vi "LCP_Scale.vi"() -> ()   [LabVIEW 2019]
uses:
  <vilib>/Instr/_visa.llb/VISA Configure Serial Port (Instr).vi
  <vilib>/Utility/file.llb/Write Delimited Spreadsheet (DBL).vi
panel:
  in  "Boolean":bool
  in  ".CSV filename":path
  in  "Weight Name":string
  out "Weight":string
  in  "stop":bool
  in  "Weights Number":i32
  in  "Ring":u8(ring) items=["Send data", "Activate calibration function", "Activate counting function", "Weighing unit selection", "Taring"]
  in  "VISA resource port":refnum<visa-resource-name>
  # ".CSV FILE NAME"
  # "VISA PORT"
  # "INSTRUCTION"
  # "REFERENCE WEIGHTS NUMBER"
  # "REFERENCE WEIGHT NAME"
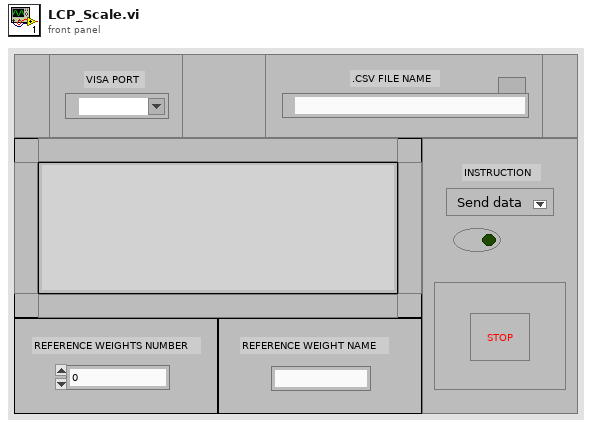
[diagram p1: front panel]
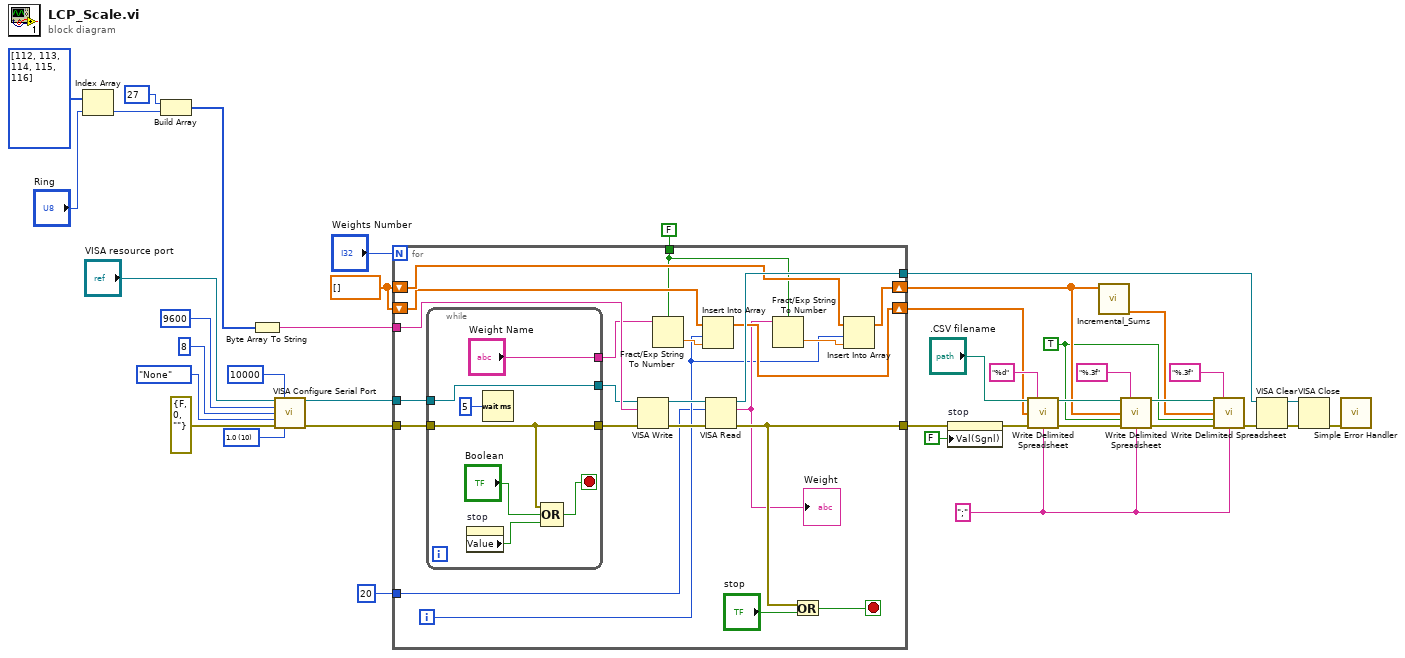
[diagram p0: block diagram]
diagram:
  w11 = TRUE ("append to file? (new file:F)")
  w8 = ";" ("delimiter (\\t)")
  w20 = dbl[] []
  w34 = u16 10 items=["1.0"=10, "1.5"=15, "2.0"=20] ("stop bits (10: 1 bit)")
  n1 = Index Array(array=u8[] [112, 113, 114, 115, 116], index="Ring") -> (element=w26:u8)
  n2 = Build Array(u8 27, w26) -> (w25:u8[])
  n3 = Byte Array To String(unsigned byte array=w25) -> (string=w24:string)
  n4 = call-poly "VISA Configure Serial Port"("VISA resource name"="VISA resource port", "timeout (10sec)"=u32 10000, "baud rate (9600)"=u32 9600, "data bits (8)"=u16 8, "parity (0:none)"=enum16{"None", "Odd", "Even", "Mark", "Space"}."None", "error in (no error)"=errorcluster {"status"=FALSE, "code"=0, "source"=""}, "stop bits (10: 1 bit)"=w34) -> ("VISA resource name out"=w33:refnum<visa-resource-name>, "error out"=w32:errorcluster)  [unwired: 7 in]
  n5 = for {
    N: "Weights Number" -> [_]
    tunnel: w24 -> [w61]
    tunnel: w33 -> [w45]
    tunnel: [w62] -> w31
    tunnel: w32 -> [w48]
    tunnel: [w58] -> w4
    shift-right: [w56] -> w13
    shift-left: w20 -> [w57]
    shift-right: [w54] -> w14
    shift-left: w20 -> [w55]
    tunnel: FALSE ("use system decimal point (T)") -> [w43]
    tunnel: u32 20 ("byte count") -> [w41]
    i -> [w42]
    stop <- w59 stop-if-true
    n6 = while {
      tunnel: w48 -> [w66]
      tunnel: [w66] -> w47
      tunnel: [w69] -> w46
      tunnel: w45 -> [w69]
      tunnel: ["Weight Name"] -> w44
      stop <- w65 stop-if-true
      n7 = property on="stop" class="Bool (strict)"() -> ("Value"=w63:bool)  [unwired: 2 in, 2 out]
      n8 = Wait (ms)(milliseconds to wait=u32 5) -> ()  [unwired: 1 out]
      n9 = Compound Arithmetic op=OR(w66, "Boolean", w63) -> (w65:bool)
    }
    n10 = VISA Write(VISA resource name=w46, write buffer=w61, error in (no error)=w47) -> (VISA resource name out=w53:refnum<visa-resource-name>, error out=w52:errorcluster)  [unwired: 1 out]
    n11 = Fract/Exp String To Number(use system decimal point (T)=w43, string=w44) -> (number=w50:dbl)  [unwired: 2 in, 1 out]
    n12 = Insert Into Array(array=w55, index=w42, new element=w50) -> (w54:dbl[])
    n13 = VISA Read(VISA resource name=w53, byte count=w41, error in (no error)=w52) -> (VISA resource name out=w62:refnum<visa-resource-name>, read buffer=w51:string, error out=w58:errorcluster)  [unwired: 1 out]
    "Weight" <- w51
    n14 = Fract/Exp String To Number(use system decimal point (T)=w43, string=w51) -> (number=w49:dbl)  [unwired: 2 in, 1 out]
    n15 = Or(x=w58, y="stop") -> (x .or. y?=w59:bool)
    n16 = Insert Into Array(array=w57, index=w42, new element=w49) -> (w56:dbl[])
  }
  n17 = property on="stop" class="Bool (strict)"(error in=w4, "Val(Sgnl)"=FALSE ("Value (Signaling)")) -> (error out=w3:errorcluster)  [unwired: 1 in, 1 out]
  n18 = call-poly <vilib>:"Write Delimited Spreadsheet.vi"("file path (dialog if empty)"=".CSV filename", "format (%.3f)"="%d", "1D data"=w14, "error in (no error)"=w3, "delimiter (\\t)"=w8) -> ("new file path (Not A Path if cancelled)"=w19:path, "error out"=w18:errorcluster)  [unwired: 9 in]
  n19 = call "Incremental_Sums.vi"("Array"=w13) -> ("output array"=w12:dbl[])  [unwired: 10 in]
  n20 = call-poly <vilib>:"Write Delimited Spreadsheet.vi"("file path (dialog if empty)"=w19, "format (%.3f)"="%.3f", "1D data"=w13, "append to file? (new file:F)"=w11, "error in (no error)"=w18, "delimiter (\\t)"=w8) -> ("new file path (Not A Path if cancelled)"=w17:path, "error out"=w16:errorcluster)  [unwired: 8 in]
  n21 = call-poly <vilib>:"Write Delimited Spreadsheet.vi"("file path (dialog if empty)"=w17, "format (%.3f)"="%.3f", "1D data"=w12, "append to file? (new file:F)"=w11, "error in (no error)"=w16, "delimiter (\\t)"=w8) -> ("error out"=w7:errorcluster)  [unwired: 8 in, 1 out]
  n22 = VISA Clear(VISA resource name=w31, error in (no error)=w7) -> (VISA resource name out=w29:refnum<visa-resource-name>, error out=w30:errorcluster)
  n23 = VISA Close(VISA resource name=w29, error in (no error)=w30) -> (error out=w6:errorcluster)
  n24 = call <vilib>:"Simple Error Handler.vi"("error in (no error)"=w6) -> ()  [unwired: 4 in, 5 out]
